vi "Finish.vi"   [LabVIEW 2020]
doc: "This VI is called just before exiting. It is expected to close I/O refnum, save collected data, etc."
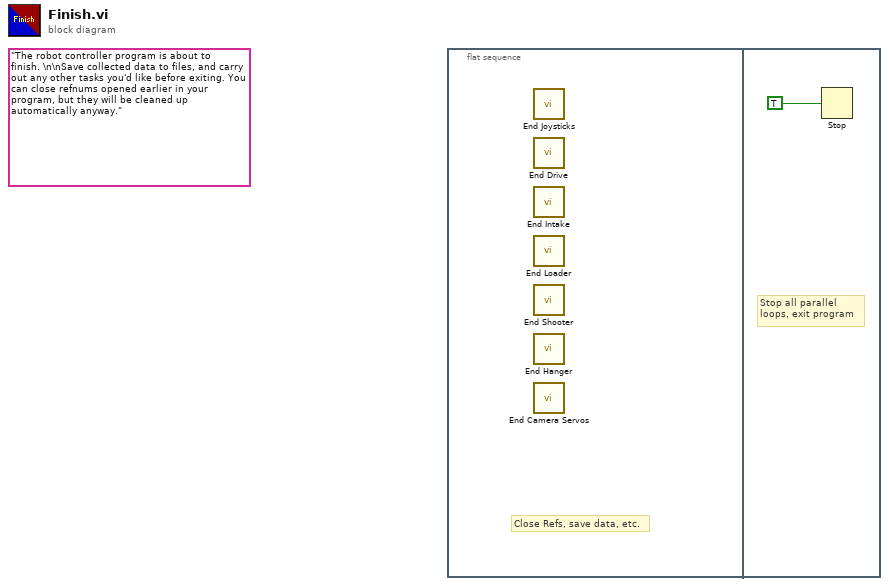
[diagram p0: block diagram]
diagram:
  (unwired) "The robot controller program is about to finish. \n\nSave collected data to files, and carry out any other tasks you'd like before exiting. You can close refnums opened earlier in your program, but they will be cleaned up automatically anyway."
  n1 = flat-sequence {
    frame #0 {
      # "Close Refs, save data, etc."
      n2 = call "End Joysticks.vi"() -> ()  [unwired: 12 in]
      n3 = call "End Drive.vi"() -> ()  [unwired: 12 in]
      n4 = call "End Intake.vi"() -> ()  [unwired: 12 in]
      n5 = call "End Loader.vi"() -> ()  [unwired: 12 in]
      n6 = call "End Shooter.vi"() -> ()  [unwired: 12 in]
      n7 = call "End Hanger.vi"() -> ()  [unwired: 12 in]
      n8 = call "End Camera Servos.vi"() -> ()  [unwired: 12 in]
    }
    frame #1 {
      # "Stop all parallel\nloops, exit program"
      n9 = Stop(stop? (T)=TRUE ("Quit")) -> ()
    }
  }
